vi "parseTopicString.vi"(8 "error in (no error)":errorcluster, 11 "Topic in":refnum<class "Topic.lvclass">) -> (0 "error out":errorcluster, 3 "Topic out":refnum<class "Topic.lvclass">)   [LabVIEW 2018, in "Topic.lvclass"]
uses:
  Topic.lvclass
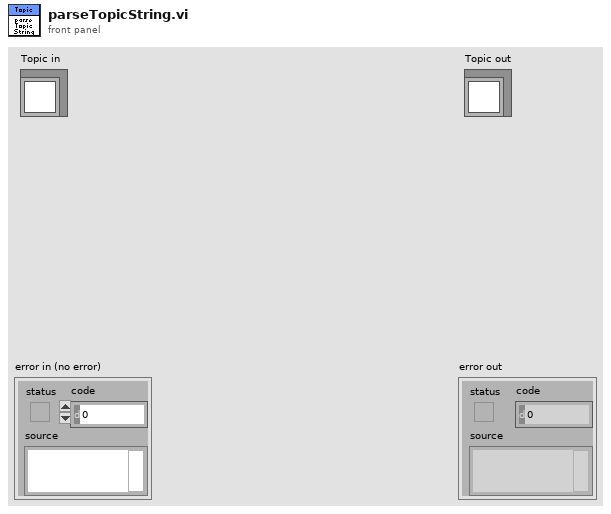
[diagram p1: front panel]
types:
  T1 = typedef "CollectionInfo.ctl" = cluster{"isArray?":bool, "arraySize":u16}
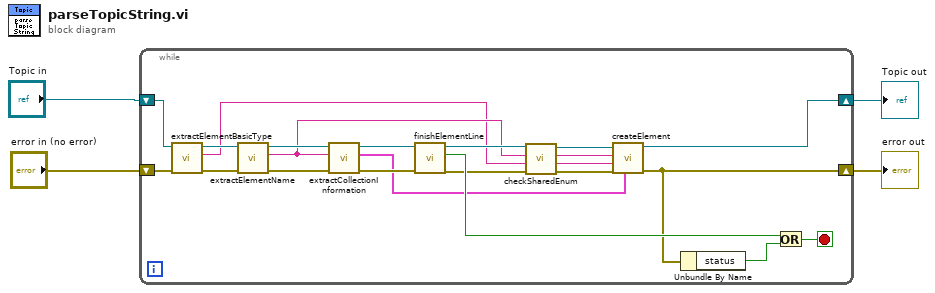
[diagram p0: block diagram]
diagram:
  n1 = while {
    shift-right: [w14] -> w3
    shift-left: "error in (no error)" -> [w20]
    shift-right: [w16] -> w1
    shift-left: "Topic in" -> [w25]
    stop <- w26 stop-if-true
    n2 = call "extractElementBasicType.vi"("error in (no error)"=w20, "Topic in"=w25) -> ("error out"=w22:errorcluster, "elementBasicType"=w7:string, "Topic out"=w24:refnum<class "Topic.lvclass">)  [unwired: 7 in]
    n3 = call "extractElementName.vi"("error in (no error)"=w22, "Topic in"=w24) -> ("error out"=w21:errorcluster, "elementName"=w8:string, "Topic out"=w23:refnum<class "Topic.lvclass">)  [unwired: 7 in]
    n4 = call "extractCollectionInformation.vi"("error in (no error)"=w21, "elementName"=w8, "Topic in"=w23) -> ("error out"=w18:errorcluster, "CollectionInfo"=w13:T1, "Topic out"=w19:refnum<class "Topic.lvclass">)  [unwired: 6 in]
    n5 = call "finishElementLine.vi"("error in (no error)"=w18, "Topic in"=w19) -> ("error out"=w9:errorcluster, "reachedEnd?"=w17:bool, "Topic out"=w12:refnum<class "Topic.lvclass">)  [unwired: 7 in]
    n6 = call "checkSharedEnum.vi"("error in (no error)"=w9, "basicType"=w7, "name"=w8, "Topic in"=w12) -> ("error out"=w10:errorcluster, "basicTypeUpdated"=w6:string, "nameDup"=w5:string, "Topic out"=w11:refnum<class "Topic.lvclass">)  [unwired: 4 in]
    n7 = call "createElement.vi"("collectionInfo"=w13, "error in (no error)"=w10, "elementBasicType"=w6, "elementName"=w5, "Topic in"=w11) -> ("error out"=w14:errorcluster, "Topic out"=w16:refnum<class "Topic.lvclass">)  [unwired: 5 in]
    n8 = Unbundle By Name(w14) -> ("status"=w15:bool)
    n9 = Or(x=w17, y=w15) -> (x .or. y?=w26:bool)
  }
  "error out" <- w3
  "Topic out" <- w1
